vi "Reset.vi"(8 "error in (no error)":errorcluster, 11 "VISA resource name":refnum<visa-resource-name>) -> (0 "error out":errorcluster, 3 "VISA resource name out":refnum<visa-resource-name>)   [LabVIEW 2011, in "Agilent 4194.lvlib"]
doc: "This function resets the instrument to a known state and sends initialization commands to the instrument that set any necessary programmatic variables such as Headers Off, Short Command form, and Data Transfer Binary to the state necessary for the operation of the instrument driver."
uses:
  <instrlib>/Agilent 4194/Agilent 4194.lvlib
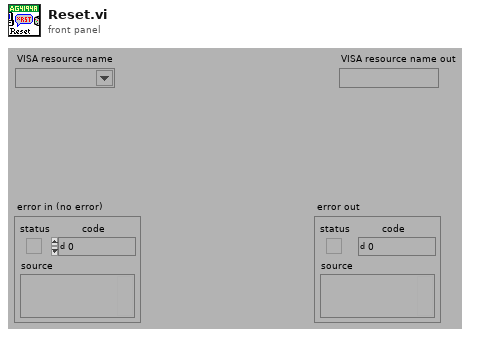
[diagram p1: front panel]
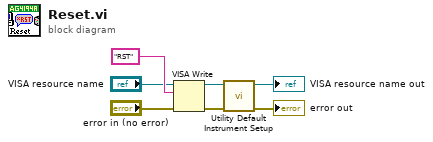
[diagram p0: block diagram]
diagram:
  n1 = VISA Write(VISA resource name="VISA resource name", write buffer="RST" ("write buffer (\"\")"), error in (no error)="error in (no error)") -> (VISA resource name out=w4:refnum<visa-resource-name>, error out=w1:errorcluster)  [unwired: 1 out]
  n2 = call <instrlib>:"Utility Default Instrument Setup.vi"("error in (no error)"=w1, "VISA resource name"=w4) -> ("error out"=→"error out":errorcluster, "VISA resource name out"=→"VISA resource name out":refnum<visa-resource-name>)  [unwired: 8 in]
